vi "1_2_TiposDeDato.vi"() -> ()   [LabVIEW 2020]
panel:
  out "Meter":dbl(knob) scale=0.0..50.0
  out "Thermometer":dbl(slide) scale=0.0..50.0
  out "Tank":dbl(slide) scale=0.0..10.0
  in  "Boolean":bool
  out "String 3":string
  out "String":string
  out "Numeric 4":dbl
  in  "Numeric":dbl
  out "Numeric 3":i32
  in  "Numeric 2":i32
  # "TIPO DE DATO INT"
  # "TIPO DE DATO DBL"
  # "TIPO DE DATO STRING"
  # "TIPO DE DATO BOOLEAN"
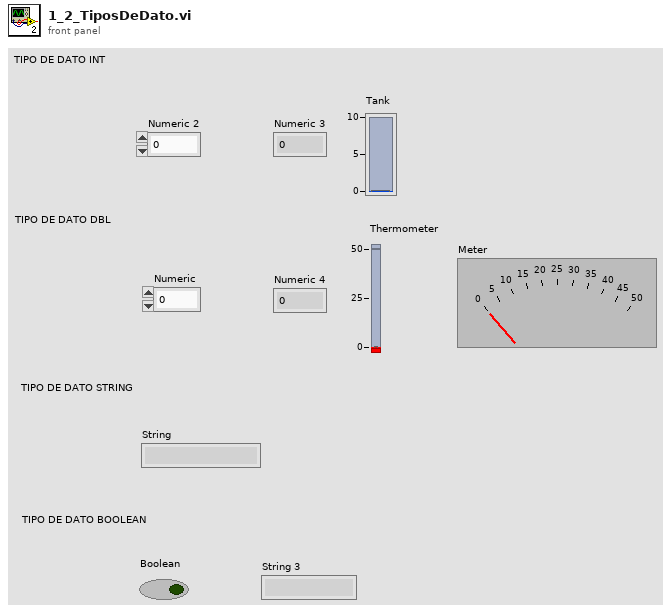
[diagram p1: front panel]
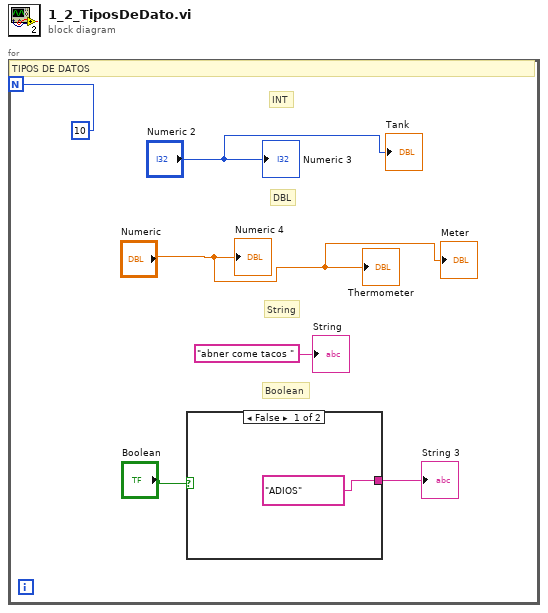
[diagram p0: block diagram]
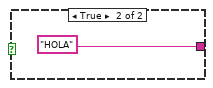
[diagram p2: hidden frame]
diagram:
  n1 = for {
    N: 10 -> [_]
    # "String"
    # "Boolean"
    # "DBL"
    # "INT"
    # "TIPOS DE DATOS"
    n2 = case shown="False" "Boolean" {
      tunnel: ["ADIOS" "HOLA"] -> w3
      frame False {
      }
      frame True {
      }
    }
    "String 3" <- w3
    "Numeric 3" <- "Numeric 2"
    "Numeric 4" <- "Numeric"
    "String" <- "abner come tacos "
    "Tank" <- "Numeric 2"
    "Thermometer" <- "Numeric"
    "Meter" <- "Numeric"
  }
